vi "digitalnumber-identify.vi"() -> ()   [LabVIEW 2015]
uses:
  <vilib>/vision/Measure.llb/Straight Edge Options.ctl
  <vilib>/vision/Measure.llb/Straight Edge Process.ctl
  <vilib>/vision/OCR.llb/IMAQ OCR Property.ctl
  <vilib>/vision/driver/NI_Vision_Acquisition_Software.lvlib
  <vilib>/vision/NI_Vision_Development_Module.lvlib
panel:
  out "识别结果":string
  out "识别图像":T1(plugin-control)
  in  "?":bool
  out "旋转后图像":T1(plugin-control)
  out "二值图像":T1(plugin-control)
  out "原始图像":T1(plugin-control)
  # "傅绮雯 5120309301\n   唐淳珏 5120309566\n      郑似兰 5120309299"
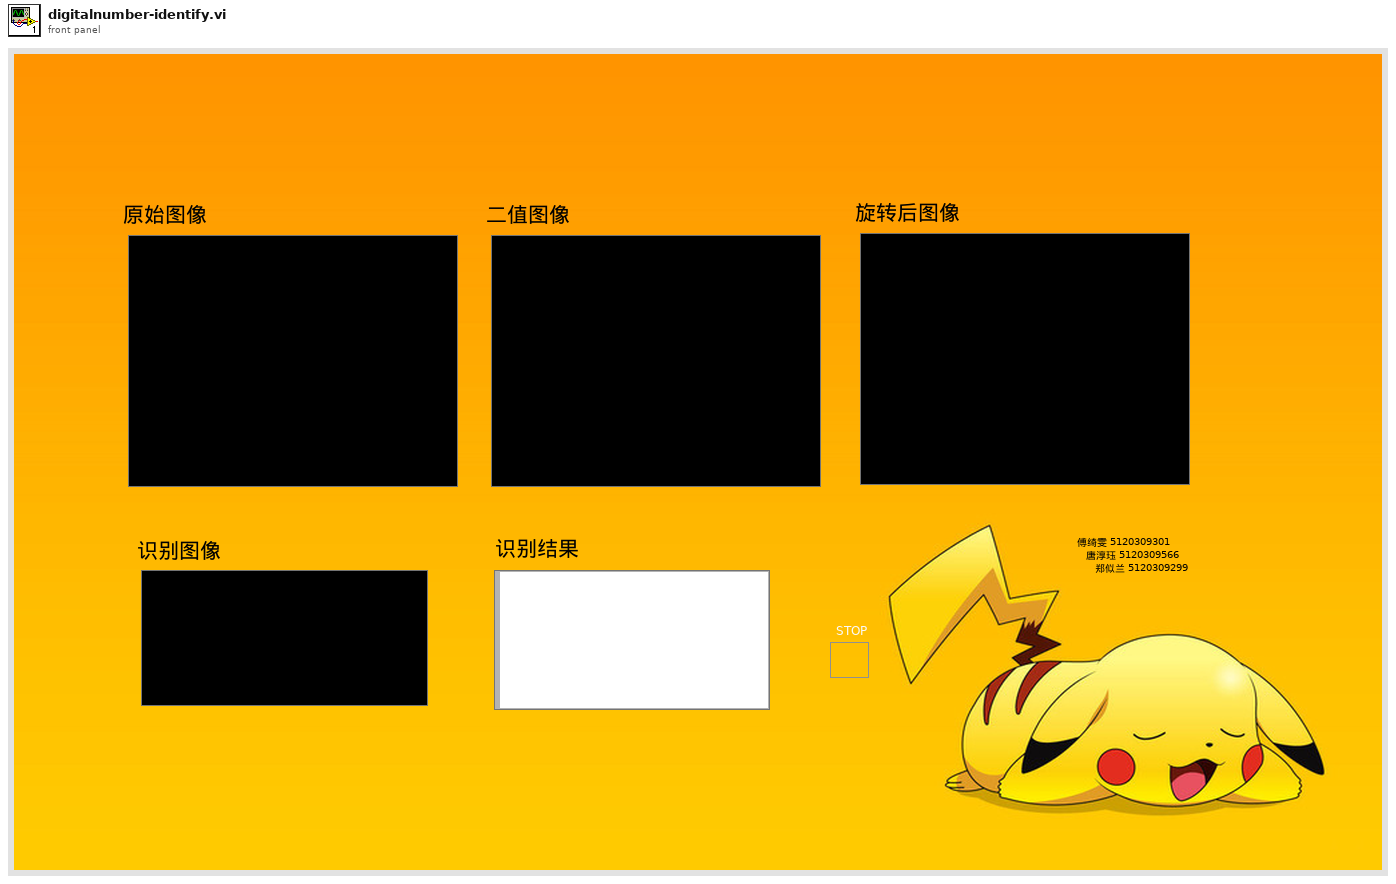
[diagram p1: front panel]
types:
  T1 = typedef "IMAQ Image.ctl" = refnum<image>
  T2 = typedef "Image Type" = u32
  T3 = typedef "IMAQdx.ctl" = refnum<k21>
  T4 = cluster{"X Size":i32, "Y Size":i32, "Order #":i32}
  T5 = cluster{"Global Rectangle":i32[], "Contours":cluster{"ID":enum32{"External", "Internal"}, "Type":u32, "Coordinates":i32[]}[]}
  T6 = typedef "Straight Edge Options.ctl" = cluster{"Number of Lines":i32, "Type":T7, "Min. Score":dbl, "Max. Score":dbl, "Orientation":dbl, "Angle Range":dbl, "Angle Tolerance":dbl, "Step Size":u32, "Min. SNR (db)":dbl, "Min. Points (%)":dbl, "Hough Iterations":i32}
  T7 = typedef "Straight Edge Process.ctl" = enum32{"First Edge Rake", "Best Edge Rake", "Hough Edge Rake", "First Edge Projection", "Best Edge Projection"}
  T8 = cluster{"Point1 (Pixels)":cluster{"X":sgl, "Y":sgl}, "Point2 (Pixels)":cluster{"X":sgl, "Y":sgl}, "Point1 (Real-World)":cluster{"X":sgl, "Y":sgl}, "Point2 (Real-World)":cluster{"X":sgl, "Y":sgl}, "Angle (Pixel)":dbl, "Angle (Real-World)":dbl, "Score":dbl, "Straightness":dbl, "Average SNR (db)":dbl, "Calibration Valid":bool}[]
  T9 = cluster{"Point1 (Pixels)":cluster{"X":sgl, "Y":sgl}, "Point2 (Pixels)":cluster{"X":sgl, "Y":sgl}, "Point1 (Real-World)":cluster{"X":sgl, "Y":sgl}, "Point2 (Real-World)":cluster{"X":sgl, "Y":sgl}, "Angle (Pixel)":dbl, "Angle (Real-World)":dbl, "Score":dbl, "Straightness":dbl, "Average SNR (db)":dbl, "Calibration Valid":bool}
  T10 = cluster{"Area":dbl, "Number of Holes":dbl, "Bounding Rect":cluster{"Left":dbl, "Top":dbl, "Right":dbl, "Bottom":dbl}, "Center of Mass":cluster{"X":dbl, "Y":dbl}, "Orientation":dbl, "Dimensions":cluster{"Width":dbl, "Height":dbl}}[]
  T11 = cluster{"Area":dbl, "Number of Holes":dbl, "Bounding Rect":cluster{"Left":dbl, "Top":dbl, "Right":dbl, "Bottom":dbl}, "Center of Mass":cluster{"X":dbl, "Y":dbl}, "Orientation":dbl, "Dimensions":cluster{"Width":dbl, "Height":dbl}}
  T12 = cluster{"Left":dbl, "Top":dbl, "Right":dbl, "Bottom":dbl}
  T13 = typedef "IMAQ OCR Property.ctl" = i32
  T14 = typedef "IMAQ OCR Session.ctl" = refnum<k1>
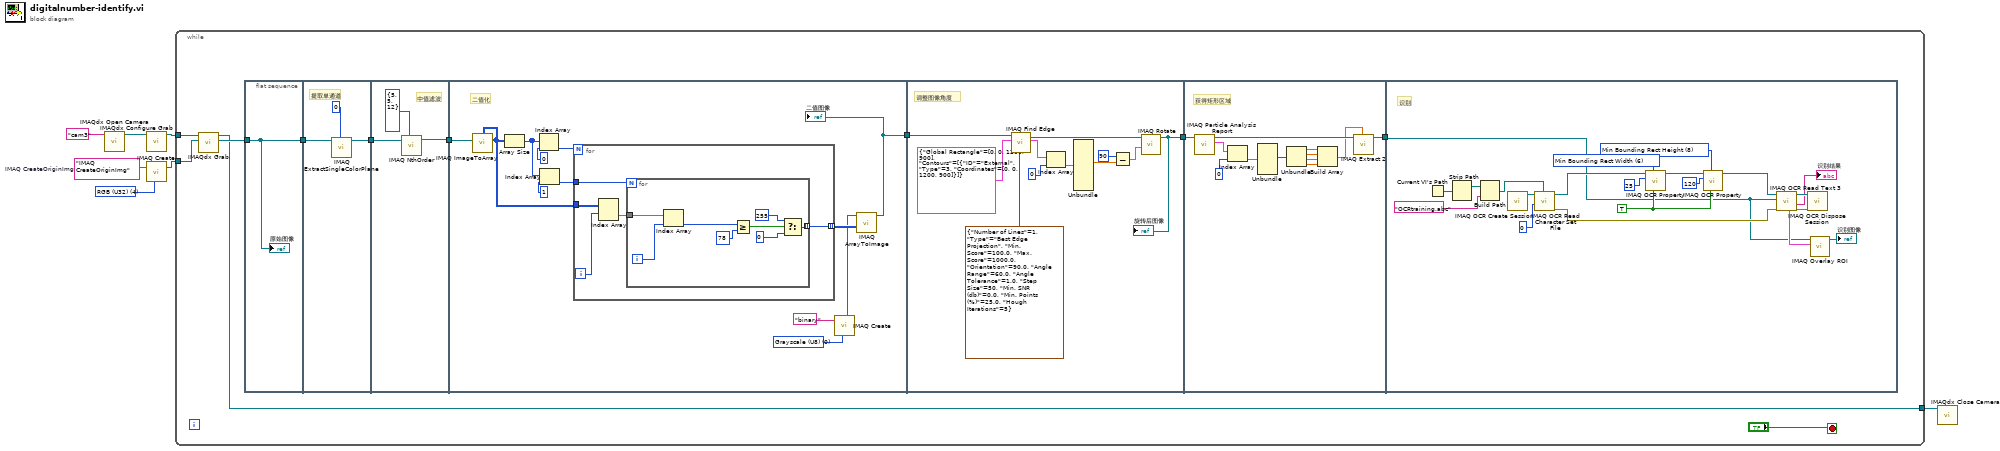
[diagram p0: block diagram]
diagram:
  w1 = T2 4 items=["Grayscale (U8)", "Grayscale (I16)", "Grayscale (SGL)", "Complex (CSG)", "RGB (U32)", "HSL (U32)", "RGB (U64)", "Grayscale (U16)"] ("Image Type")
  w5 = "IMAQ CreateOriginImg"  # IMAQ CreateOriginImg
  n1 = call <vilib>:"IMAQdx Open Camera.vi"("Session In"="cam3") -> ("Session Out"=w7:T3)  [unwired: 9 in, 1 out]
  n2 = call <vilib>:"IMAQdx Configure Grab.vi"("Session In"=w7) -> ("Session Out"=w4:T3)  [unwired: 9 in, 1 out]
  n3 = call "IMAQ Create"("Image Name"=w5, "Image Type"=w1) -> ("New Image"=w3:T1)  [unwired: 3 in, 1 out]
  n4 = while {
    tunnel: w4 -> [w18]
    tunnel: w3 -> [w17]
    tunnel: [w9] -> w2
    stop <- "?" stop-if-true
    n5 = call <vilib>:"IMAQdx Grab.vi"("Image In"=w17, "Session In"=w18) -> ("Image Out"=w14:T1, "Session Out"=w9:T3)  [unwired: 6 in, 2 out]
    n6 = flat-sequence {
      tunnel: w14 -> [w19]
      tunnel: [w19] -> w13
      tunnel: [w20] -> w11
      tunnel: w13 -> [w21]
      tunnel: w11 -> [w24]
      tunnel: [w23] -> w10
      tunnel: w10 -> [w28]
      tunnel: [w26] -> w12
      tunnel: [w53] -> w15
      tunnel: w12 -> [w56]
      tunnel: [w62] -> w16
      tunnel: w15 -> [w67]
      tunnel: w16 -> [w74]
      frame #0 {
        "原始图像" <- w19
      }
      frame #1 {
        # "提取单通道"
        n7 = call "IMAQ ExtractSingleColorPlane"("Color Plane"=0, "Image Src"=w21) -> ("Image Dst Out"=w20:T1)  [unwired: 8 in, 1 out]
      }
      frame #2 {
        # "中值滤波"
        n8 = call "IMAQ NthOrder"("Image Src"=w24, "Size & Order #"=T4 {"X Size"=5, "Y Size"=5, "Order #"=12}) -> ("Image Dst Out"=w23:T1)  [unwired: 3 in, 3 out]
      }
      frame #3 {
        w29 = T2 0 items=["Grayscale (U8)", "Grayscale (I16)", "Grayscale (SGL)", "Complex (CSG)", "RGB (U32)", "HSL (U32)", "RGB (U64)", "Grayscale (U16)"] ("Image Type")
        # "二值化"
        n9 = call "IMAQ ImageToArray"("Image"=w28) -> ("Image Pixels (U8)"=w31:u8[][])  [unwired: 3 in, 4 out]
        n10 = Array Size(array=w31) -> (size(s)=w33:i32[])
        n11 = Index Array(array=w33, index=0) -> (element=w32:i32)
        n12 = Index Array(array=w33, index=1) -> (element=w35:i32)
        n13 = for {
          N: w32 -> [_]
          tunnel: w35 -> [w38]
          tunnel: [w42] -> w34 mode=indexing
          tunnel: w31 -> [w39]
          i -> [w41]
          n14 = Index Array ("索引数组")(array=w39, index (row)=w41) -> (element=w40:u8[])  [unwired: 1 in]
          n15 = for {
            N: w38 -> [_]
            tunnel: [w46] -> w42 mode=indexing
            tunnel: w40 -> [w45]
            i -> [w50]
            n16 = Index Array(array=w45, index=w50) -> (element=w44:u8)
            n17 = Greater Or Equal?(x=w44, y=u8 78) -> (x >= y?=w47:bool)
            n18 = Select(t=255, s=w47, f=0) -> (s? t:f=w46:i32)
          }
        }
        n19 = call "IMAQ Create"("Image Name"="binary", "Image Type"=w29) -> ("New Image"=w27:T1)  [unwired: 3 in, 1 out]
        n20 = call "IMAQ ArrayToImage"("Image Pixels (U8)"=w34, "Image"=w27) -> ("Image Out"=w26:T1)  [unwired: 8 in, 1 out]
        "二值图像" <- w26
      }
      frame #4 {
        # "调整图像角度"
        n21 = call "IMAQ Find Edge"("Line Fit Options"=T6 {"Number of Lines"=1, "Type"=enum."Best Edge Projection", "Min. Score"=100.0, "Max. Score"=1000.0, "Orientation"=90.0, "Angle Range"=60.0, "Angle Tolerance"=1.0, "Step Size"=50, "Min. SNR (db)"=0.0, "Min. Points (%)"=25.0, "Hough Iterations"=5}, "ROI Descriptor"=T5 {"Global Rectangle"=[0, 0, 1200, 900], "Contours"=[{"ID"=enum."External", "Type"=3, "Coordinates"=[0, 0, 1200, 900]}]}, "Image"=w56) -> ("Straight Edges"=w54:T8, "Image Out"=w55:T1)  [unwired: 5 in, 2 out]
        n22 = Index Array(array=w54, index=0) -> (element=w61:T9)
        n23 = Unbundle(w61) -> ("Angle (Pixel)"=w57:dbl)  [unwired: 9 out]
        n24 = Subtract(x=90, y=w57) -> (x-y=w58:dbl)
        n25 = call "IMAQ Rotate"("Angle (degrees)"=w58, "Image Src"=w55) -> ("Image Dst Out"=w53:T1)  [unwired: 8 in, 1 out]
        "旋转后图像" <- w53
      }
      frame #5 {
        # "获得矩形区域"
        n26 = call "IMAQ Particle Analysis Report"("Image"=w67) -> ("Particle Reports (Pixels)"=w71:T10, "Image Out (duplicate)"=w73:T1)  [unwired: 5 in, 4 out]
        n27 = Index Array(array=w71, index=0) -> (element=w69:T11)
        n28 = Unbundle(w69) -> ("Bounding Rect"=w68:T12)  [unwired: 5 out]
        n29 = Unbundle(w68) -> ("Left"=w66:dbl, "Top"=w65:dbl, "Right"=w64:dbl, "Bottom"=w63:dbl)
        n30 = Build Array(w66, w65, w64, w63) -> (w72:dbl[])
        n31 = call "IMAQ Extract 2"("Optional Rectangle"=w72, "Image Src"=w73) -> ("Image Dst Out"=w62:T1)  [unwired: 8 in, 1 out]
      }
      frame #6 {
        w80 = T13 8 items=["Acceptance Level", "Min Char Size", "Max Char Size", "Min Char Spacing", "Max Horiz Element Spacing", "Max Vert Element Spacing", "Min Bounding Rect Width", "Max Bounding Rect Width", "Min Bounding Rect Height", "Max Bounding Rect Height", "Read Strategy", "Aspect Ratio", "Number Of Erosions", "Read Resolution", "Size of Char Set", "Substitution Character", "Remove Particles Touching ROI", "Auto Split"] ("Property")
        w81 = T13 6 items=["Acceptance Level", "Min Char Size", "Max Char Size", "Min Char Spacing", "Max Horiz Element Spacing", "Max Vert Element Spacing", "Min Bounding Rect Width", "Max Bounding Rect Width", "Min Bounding Rect Height", "Max Bounding Rect Height", "Read Strategy", "Aspect Ratio", "Number Of Erosions", "Read Resolution", "Size of Char Set", "Substitution Character", "Remove Particles Touching ROI", "Auto Split"] ("Property")
        w79 = TRUE
        # "识别"
        n32 = Current VI's Path() -> (path=w92:path)
        n33 = Strip Path(path=w92) -> (stripped path=w91:path)  [unwired: 1 out]
        n34 = Build Path(base path=w91, name or relative path="OCRtraining.abc") -> (appended path=w93:path)
        n35 = call "IMAQ OCR Create Session"() -> ("IMAQ OCR Session"=w86:T14)  [unwired: 10 in, 1 out]
        n36 = call "IMAQ OCR Read Character Set File"("File Path"=w93, "Read Options"=0, "IMAQ OCR Session"=w86) -> ("error out"=w89:errorcluster, "IMAQ OCR Session (dup)"=w77:T14)  [unwired: 6 in, 1 out]
        n37 = call-poly "IMAQ OCR Property"("Get/Set (True: Set)"=w79, "Property"=w81, "Property Value"=25, "IMAQ OCR Session"=w77) -> ("IMAQ OCR Session (dup)"=w84:T14)  [unwired: 5 in, 2 out]
        n38 = call-poly "IMAQ OCR Property"("Get/Set (True: Set)"=w79, "Property"=w80, "Property Value"=120, "IMAQ OCR Session"=w84) -> ("IMAQ OCR Session (dup)"=w78:T14)  [unwired: 5 in, 2 out]
        n39 = call "IMAQ OCR Read Text 3"("error in (no error)"=w89, "Image"=w74, "IMAQ OCR Session"=w78) -> ("error out"=w88:errorcluster, "Read String"=→"识别结果":string, "IMAQ OCR Session (dup)"=w90:T14, "ROI Bounding Characters"=w75:T5)  [unwired: 3 in, 2 out]
        n40 = call "IMAQ OCR Dispose Session"("error in (no error)"=w88, "IMAQ OCR Session"=w90) -> ()  [unwired: 9 in, 1 out]
        n41 = call "IMAQ Overlay ROI"("ROI Descriptor"=w75, "Image"=w74) -> ("Image Out"=→"识别图像":T1)  [unwired: 4 in, 5 out]
      }
    }
  }
  n42 = call <vilib>:"IMAQdx Close Camera.vi"("Session In"=w2) -> ()  [unwired: 10 in, 1 out]
